vi "GetLIDAR.vi"(1 "Roll (deg)":dbl, 2 "Pitch (deg)":dbl, 3 "Raw Horizontal Offset (in)":dbl) -> (0 "LIDAR Distance to Target (in)":dbl)   [LabVIEW 2019]
doc: "This VI converts the raw LIDAR signal into a range in inches and is based on code from FRC 3504. https://www.andymark.com/products/lidar-lite-3"
uses:
  refnums.vi
  GRNF_DIC.vi
  sensors.vi
  constants.vi
panel:
  in  "Maximum Pointing Error (deg)":dbl=5.0
  in  "Calibration Offset (in)":dbl=10.0
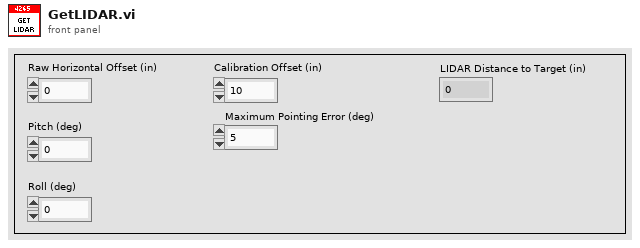
[diagram p1: front panel]
types:
  T1 = typedef "WPI_CounterDevRef.ctl" = cluster{"DevStatus":errorcluster, "CntIndex":T2}
  T2 = typedef "FPGA_CounterCtrSystemIndex.ctl" = enum8{"Ctr 0", "Ctr 1", "Ctr 2", "Ctr 3", "Ctr 4", "Ctr 5", "Ctr 6", "Ctr 7", "Invalid"}
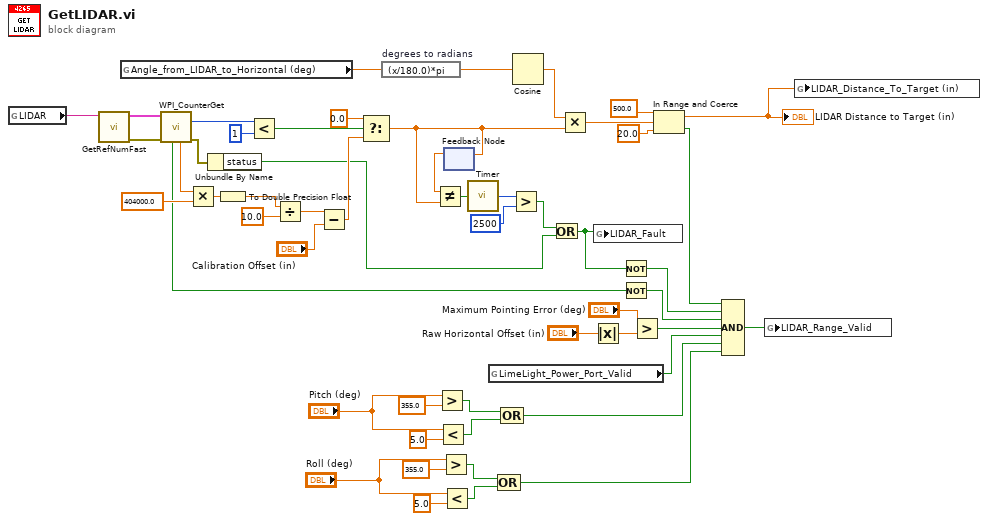
[diagram p0: block diagram]
diagram:
  n1 = global read "refnums.vi" "LIDAR"() -> (w41:string)
  n2 = call-poly "GetRefNumFast.vi"("RefNum Name"=w41) -> ("Error"=w39:errorcluster, "Device Reference"=w40:T1)  [unwired: 5 in]
  n3 = global read "constants.vi" "Angle_from_LIDAR_to_Horizontal (deg)"() -> (w9:dbl)
  n4 = call <vilib>:"WPI_CounterGet.vi"("error in (no error)"=w39, "CounterDevRef in"=w40) -> ("error out"=w14:errorcluster, "Value"=w50:i32, "Period (sec)"=w43:dbl, "Stopped"=w15:bool)  [unwired: 4 in, 2 out]
  n5 = Multiply(x=w43, y=404000.0) -> (x*y=w49:dbl)
  n6 = Unbundle By Name(w14) -> ("status"=w2:bool)
  n7 = To Double Precision Float(number=w49) -> (double precision float=w48:dbl)
  n8 = Less?(x=w50, y=1) -> (x < y?=w53:bool)
  n9 = Divide(x=w48, y=10.0) -> (x/y=w46:dbl)
  n10 = Subtract(x=w46, y="Calibration Offset (in)") -> (x-y=w44:dbl)
  n11 = Select(t=0.0, s=w53, f=w44) -> (s? t:f=w8:dbl)
  n12 = expression code="(x/180.0)*pi" "degrees to radians"(w9) -> (w10:dbl)
  n13 = Greater?(x="Pitch (deg)", y=355.0) -> (0:w28:bool)
  n14 = Less?(x="Pitch (deg)", y=5.0) -> (x < y?=w27:bool)
  n15 = Greater?(x="Roll (deg)", y=355.0) -> (0:w24:bool)
  n16 = Less?(x="Roll (deg)", y=5.0) -> (x < y?=w23:bool)
  n17 = feedback-in #1(w8) -> ()
  n18 = feedback #1() -> (w7:dbl)  [unwired: 1 in]
  n19 = Not Equal?(x=w7, y=w8) -> (x != y?=w6:bool)
  n20 = call "Timer.vi"("Reset Timer"=w6) -> ("Time (ms)"=w5:u32)
  n21 = global read "sensors.vi" "LimeLight_Power_Port_Valid"() -> (w34:bool)
  n22 = Compound Arithmetic op=OR(w24, w23) -> (w19:bool)
  n23 = Compound Arithmetic op=OR(w28, w27) -> (w20:bool)
  n24 = Greater?(x=w5, y=u32 2500) -> (0:w3:bool)
  n25 = Cosine(x=w10) -> (cos(x)=w12:dbl)
  n26 = Or(x=w3, y=w2) -> (x .or. y?=w1:bool)
  n27 = Multiply(x=w12, y=w8) -> (x*y=w11:dbl)
  n28 = Absolute Value(x="Raw Horizontal Offset (in)") -> (abs(x)=w37:dbl)
  n29 = global write "sensors.vi" "LIDAR_Fault"(w1) -> ()
  n30 = Not(x=w1) -> (.not. x?=w13:bool)
  n31 = Not(x=w15) -> (.not. x?=w16:bool)
  n32 = Greater?(x="Maximum Pointing Error (deg)", y=w37) -> (0:w35:bool)
  n33 = In Range and Coerce(upper limit=500.0, x=w11, lower limit=20.0 ("x")) -> (coerced(x)=w31:dbl, In Range?=w17:bool)
  "LIDAR Distance to Target (in)" <- w31
  n34 = Compound Arithmetic op=AND(w17, w13, w16, w35, w34, w20, w19) -> (w18:bool)
  n35 = global write "sensors.vi" "LIDAR_Range_Valid"(w18) -> ()
  n36 = global write "sensors.vi" "LIDAR_Distance_To_Target (in)"(w31) -> ()
